vi "Parse Instrumnet Info for User Display.vi"(8 "error in (no error)":errorcluster, 10 "Inst Info only output":string[][](array[string]), 11 "Station in":refnum<class "Station.lvclass">) -> (0 "error out":errorcluster, 3 "Station out":refnum<class "Station.lvclass">)   [LabVIEW 2018, in "Station.lvclass"]
uses:
  Station.lvclass
  Station.lvclass/Station.ctl
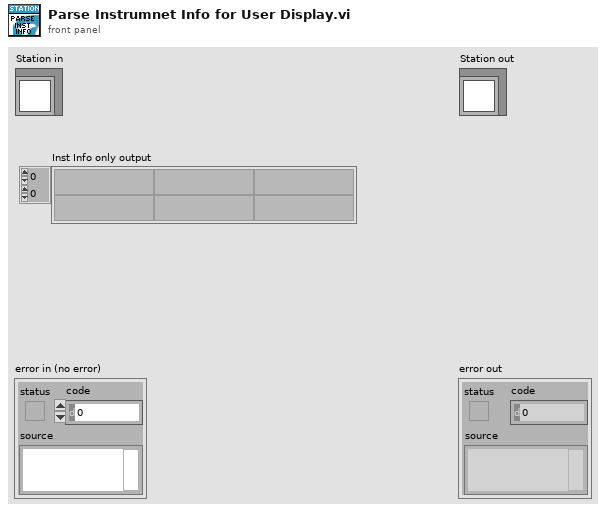
[diagram p1: front panel]
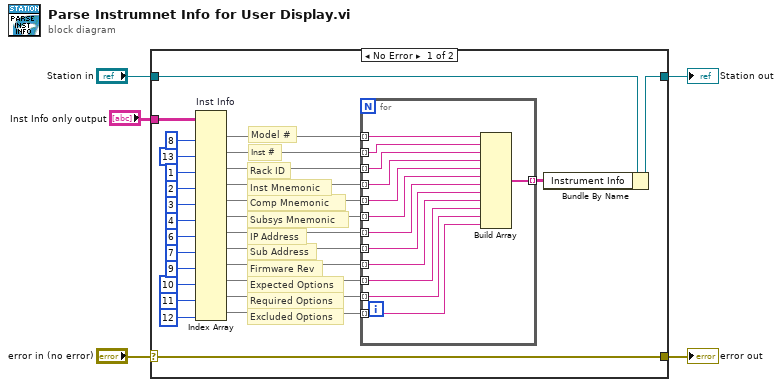
[diagram p0: block diagram]
diagram:
  n1 = case shown="No Error" "error in (no error)" {
    selector: "error in (no error)" -> [w33 w49]
    tunnel: [w33 w49] -> w3
    tunnel: "Inst Info only output" -> [w32 _]
    tunnel: "Station in" -> [w8 w48]
    tunnel: [w7 w48] -> w1
    frame No Error {
      # "Inst #"
      # "Comp Mnemonic"
      # "Subsys Mnemonic"
      # "Inst Mnemonic"
      # "Rack ID"
      # "Excluded Options"
      # "Required Options"
      # "Expected Options"
      # "Firmware Rev"
      # "Model #"
      # "Sub Address"
      # "IP Address"
      n2 = Index Array "Inst Info"(array=w32, index (col) #1=8 ("disabled index (col)"), index (col) #2=13 ("index (col)"), index (col) #3=1 ("index (col)"), index (col) #4=2 ("index (col)"), index (col) #5=3 ("index (col)"), index (col) #6=4 ("index (col)"), index (col) #7=6 ("index (col)"), index (col) #8=7 ("index (col)"), index (col) #9=9 ("index (col)"), index (col) #10=10 ("index (col)"), index (col) #11=11 ("index (col)"), index (col) #12=12 ("index (col)")) -> (element #1=w31:string[], element #2=w30:string[], element #3=w29:string[], element #4=w28:string[], element #5=w24:string[], element #6=w23:string[], element #7=w22:string[], element #8=w21:string[], element #9=w20:string[], element #10=w19:string[], element #11=w18:string[], element #12=w9:string[])  [unwired: 12 in]
      n3 = for {
        tunnel: w31 -> [w47] mode=indexing
        tunnel: w30 -> [w46] mode=indexing
        tunnel: w29 -> [w45] mode=indexing
        tunnel: w28 -> [w44] mode=indexing
        tunnel: w24 -> [w43] mode=indexing
        tunnel: w23 -> [w42] mode=indexing
        tunnel: w22 -> [w41] mode=indexing
        tunnel: w21 -> [w40] mode=indexing
        tunnel: w20 -> [w39] mode=indexing
        tunnel: w19 -> [w38] mode=indexing
        tunnel: w18 -> [w37] mode=indexing
        tunnel: w9 -> [w36] mode=indexing
        tunnel: [w35] -> w6 mode=indexing
        n4 = Build Array(w47, w46, w45, w44, w43, w42, w41, w40, w39, w38, w37, w36) -> (w35:string[])
      }
      n5 = Bundle By Name(cluster=w8, "Instrument Info"=w6) -> (w7:refnum<class "Station.lvclass">)
    }
    frame Error {
    }
  }
  "error out" <- w3
  "Station out" <- w1
